vi "Nano-drive set using NI.vi"(5 "axis":u8 caption="1=x, 2=y, 3= z", 7 "0 - 10V":ext format="%.7f") -> ()   [LabVIEW 2011]
doc: "Low-level routine to do a one-axis move of the Mad City piezo stage. Modified 9/24/04 to correct bug in Mad City's version that improperly encoded the voltage into a 20 bit number."
uses:
  <vilib>/DAQmx/write.llb/DAQmx Write (Digital U32 1Chan 1Samp).vi
  <vilib>/DAQmx/write.llb/DAQmx Write (Digital U8 1Chan 1Samp).vi
  <vilib>/DAQmx/create/channels.llb/DAQmx Create Channel (DO-Digital Output).vi
  <vilib>/DAQmx/miscellaneous.llb/DAQmx Fill In Error Info.vi
panel:
  out "port 0 lsb":bool[](array[boolean])
  out "port 1":bool[](array[boolean])
  out "port 2 msb":bool[](array[boolean])
  # "For TTL mad city stage only"
  # "LSB"
  # "MSB"
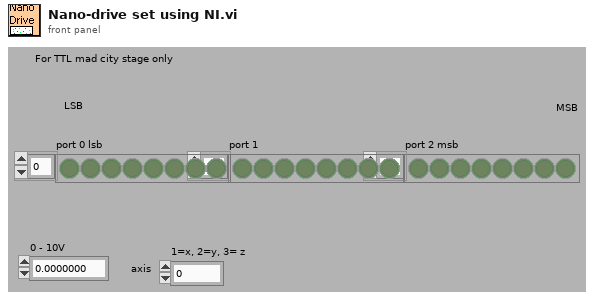
[diagram p1: front panel]
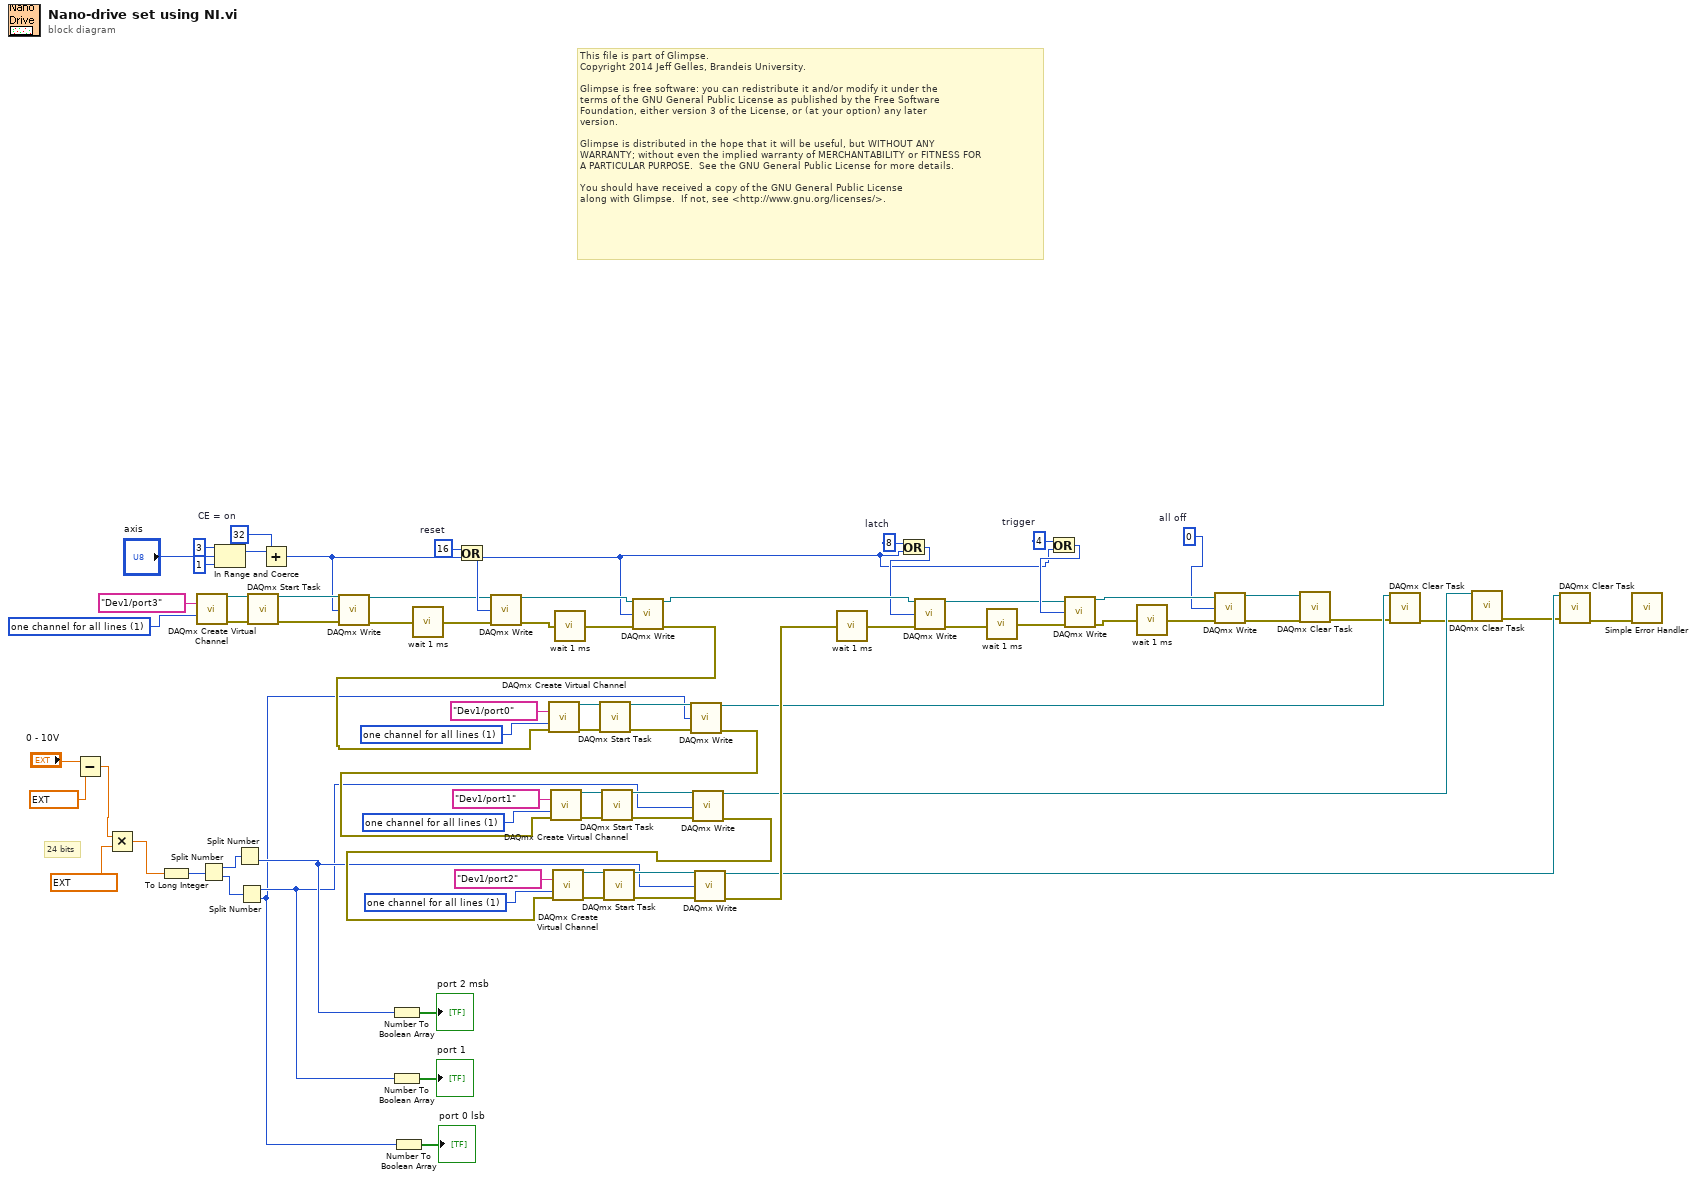
[diagram p0: block diagram]
diagram:
  w20 = u8 0  # all off
  w27 = u8 4  # trigger
  w30 = u8 8  # latch
  w42 = 1 items=["one channel for each line", "one channel for all lines"] ("line grouping")
  w53 = 1 items=["one channel for each line", "one channel for all lines"] ("line grouping")
  w54 = 1 items=["one channel for each line", "one channel for all lines"] ("line grouping")
  w67 = u8 16  # reset
  w72 = u8 32  # CE = on
  w78 = 1 items=["one channel for each line", "one channel for all lines"] ("line grouping")
  # "This file is part of Glimpse. \nCopyright 2014 Jeff Gelles, Brandeis University.    \n\nGlimpse is free software: you can redistribute it and/or modify it under the \nterms of the GNU General Public License as published by the Free Software \nFoundation, either version 3 of the License, or (at your option) any later \nversion.\n\nGlimpse is distributed in the hope that it will be useful, but WITHOUT ANY \nWARRANTY; without even the implied warranty of MERCHANTABILITY or FITNESS FOR \nA PARTICULAR PURPOSE.  See the GNU General Public License for more details.\n\nYou should have received a copy of the GNU General Public License\nalong with Glimpse.  If not, see <http://www.gnu.org/licenses/>."
  # "24 bits"
  n1 = Subtract(x="0 - 10V", y=ext 5.0) -> (x-y=w40:ext)
  n2 = Multiply(x=w40, y=ext 1677721.6) -> (x*y=w41:ext)
  n3 = To Long Integer(number=w41) -> (32bit integer=w7:i32)
  n4 = call-poly <vilib>:"DAQmx Create Virtual Channel.vi"("lines"=tag "Dev1/port3", "line grouping"=w78) -> ("task out"=w75:refnum<k21>, "error out"=w76:errorcluster)  [unwired: 3 in, 9 out]
  n5 = Split Number(x=w7) -> (hi(x)=w8:u16, lo(x)=w9:u16)
  n6 = In Range and Coerce(upper limit=u8 3, x="axis", lower limit=u8 1) -> (coerced(x)=w71:u8)  [unwired: 1 out]
  n7 = Split Number(x=w8) -> (lo(x)=w3:u8)  [unwired: 1 out]
  n8 = Split Number(x=w9) -> (hi(x)=w2:u8, lo(x)=w1:u8)
  n9 = call <vilib>:"DAQmx Start Task.vi"("task/channels in"=w75, "error in"=w76) -> ("task out"=w74:refnum<k21>, "error out"=w73:errorcluster)  [unwired: 12 out]
  n10 = Add(x=w71, y=w72) -> (x+y=w19:u8)
  n11 = call-poly <vilib>:"DAQmx Write.vi"("task/channels in"=w74, "data"=w19, "error in"=w73) -> ("task out"=w61:refnum<k21>, "error out"=w65:errorcluster)  [unwired: 1 in, 10 out]
  n12 = Number To Boolean Array(number=w3) -> (Boolean array=→"port 2 msb":bool[])
  n13 = Number To Boolean Array(number=w2) -> (Boolean array=→"port 1":bool[])
  n14 = Number To Boolean Array(number=w1) -> (Boolean array=→"port 0 lsb":bool[])
  n15 = call "wait 1 ms.vi"("error in"=w65) -> ("error  out"=w64:errorcluster)
  n16 = Or(x=w67, y=w19) -> (x .or. y?=w66:u8)
  n17 = call-poly <vilib>:"DAQmx Write.vi"("task/channels in"=w61, "data"=w66, "error in"=w64) -> ("task out"=w60:refnum<k21>, "error out"=w62:errorcluster)  [unwired: 2 in, 9 out]
  n18 = call "wait 1 ms.vi"("error in"=w62) -> ("error  out"=w63:errorcluster)
  n19 = call-poly <vilib>:"DAQmx Write.vi"("task/channels in"=w60, "data"=w19, "error in"=w63) -> ("task out"=w31:refnum<k21>, "error out"=w36:errorcluster)  [unwired: 1 in, 10 out]
  n20 = call-poly <vilib>:"DAQmx Create Virtual Channel.vi"("lines"=tag "Dev1/port0", "line grouping"=w54, "error in"=w36) -> ("task out"=w57:refnum<k21>, "error out"=w56:errorcluster)  [unwired: 4 in, 7 out]
  n21 = call <vilib>:"DAQmx Start Task.vi"("task/channels in"=w57, "error in"=w56) -> ("task out"=w58:refnum<k21>, "error out"=w59:errorcluster)  [unwired: 12 out]
  n22 = call-poly <vilib>:"DAQmx Write.vi"("task/channels in"=w58, "data"=w1, "error in"=w59) -> ("task out"=w17:refnum<k21>, "error out"=w35:errorcluster)  [unwired: 1 in, 10 out]
  n23 = call-poly <vilib>:"DAQmx Create Virtual Channel.vi"("lines"=tag "Dev1/port1", "line grouping"=w53, "error in"=w35) -> ("task out"=w50:refnum<k21>, "error out"=w51:errorcluster)  [unwired: 4 in, 7 out]
  n24 = call <vilib>:"DAQmx Start Task.vi"("task/channels in"=w50, "error in"=w51) -> ("task out"=w49:refnum<k21>, "error out"=w48:errorcluster)  [unwired: 12 out]
  n25 = call-poly <vilib>:"DAQmx Write.vi"("task/channels in"=w49, "data"=w2, "error in"=w48) -> ("task out"=w16:refnum<k21>, "error out"=w34:errorcluster)  [unwired: 1 in, 10 out]
  n26 = call-poly <vilib>:"DAQmx Create Virtual Channel.vi"("lines"=tag "Dev1/port2", "line grouping"=w42, "error in"=w34) -> ("task out"=w45:refnum<k21>, "error out"=w44:errorcluster)  [unwired: 4 in, 7 out]
  n27 = call <vilib>:"DAQmx Start Task.vi"("task/channels in"=w45, "error in"=w44) -> ("task out"=w46:refnum<k21>, "error out"=w47:errorcluster)  [unwired: 12 out]
  n28 = call-poly <vilib>:"DAQmx Write.vi"("task/channels in"=w46, "data"=w3, "error in"=w47) -> ("task out"=w15:refnum<k21>, "error out"=w32:errorcluster)  [unwired: 1 in, 10 out]
  n29 = call "wait 1 ms.vi"("error in"=w32) -> ("error  out"=w33:errorcluster)
  n30 = Or(x=w30, y=w19) -> (x .or. y?=w29:u8)
  n31 = call-poly <vilib>:"DAQmx Write.vi"("task/channels in"=w31, "data"=w29, "error in"=w33) -> ("task out"=w24:refnum<k21>, "error out"=w25:errorcluster)  [unwired: 1 in, 10 out]
  n32 = call "wait 1 ms.vi"("error in"=w25) -> ("error  out"=w26:errorcluster)
  n33 = Or(x=w27, y=w19) -> (x .or. y?=w28:u8)
  n34 = call-poly <vilib>:"DAQmx Write.vi"("task/channels in"=w24, "data"=w28, "error in"=w26) -> ("task out"=w22:refnum<k21>, "error out"=w21:errorcluster)  [unwired: 1 in, 10 out]
  n35 = call "wait 1 ms.vi"("error in"=w21) -> ("error  out"=w23:errorcluster)
  n36 = call-poly <vilib>:"DAQmx Write.vi"("task/channels in"=w22, "data"=w20, "error in"=w23) -> ("task out"=w18:refnum<k21>, "error out"=w14:errorcluster)  [unwired: 1 in, 10 out]
  n37 = call <vilib>:"DAQmx Clear Task.vi"("task in"=w18, "error in"=w14) -> ("error out"=w13:errorcluster)  [unwired: 13 out]
  n38 = call <vilib>:"DAQmx Clear Task.vi"("task in"=w17, "error in"=w13) -> ("error out"=w12:errorcluster)  [unwired: 13 out]
  n39 = call <vilib>:"DAQmx Clear Task.vi"("task in"=w16, "error in"=w12) -> ("error out"=w11:errorcluster)  [unwired: 13 out]
  n40 = call <vilib>:"DAQmx Clear Task.vi"("task in"=w15, "error in"=w11) -> ("error out"=w10:errorcluster)  [unwired: 13 out]
  n41 = call <vilib>:"Simple Error Handler.vi"("error in (no error)"=w10) -> ()  [unwired: 1 in, 8 out]
